vi "execute.vi"(10 "task token":refnum<class "null task token.lvclass">, 11 "noncancellable wait in":refnum<class "noncancellable wait.lvclass">) -> (3 "result":refnum<class "result.lvclass">)   [LabVIEW 2013, in "noncancellable wait.lvclass"]
uses:
  noncancellable wait.lvclass
  result/result.lvclass
  task token/null task token.lvclass
  action/action.lvclass/action.ctl
  action/action.lvclass
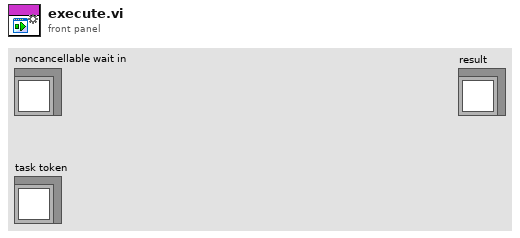
[diagram p1: front panel]
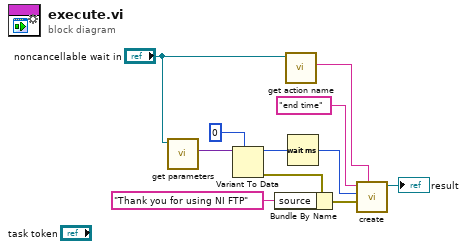
[diagram p0: block diagram]
diagram:
  n1 = call "get parameters.vi"("action in"="noncancellable wait in") -> ("parameters"=w11:variant)  [unwired: 9 in, 1 out]
  n2 = Variant To Data(type=u32 0 ("milliseconds to wait"), Variant=w11) -> (data=w2:u32, error out=w9:errorcluster)  [unwired: 1 in]
  n3 = Bundle By Name(cluster=w9, "source"="Thank you for using NI FTP") -> (w6:errorcluster)
  n4 = call "get action name.vi"("action in"="noncancellable wait in") -> ("action name"=w7:string)  [unwired: 9 in, 1 out]
  n5 = Wait (ms)(milliseconds to wait=w2) -> (millisecond timer value=w1:u32)
  n6 = call "create.vi"("generating action"=w7, "error"=w6, "data"=w1, "data ID"="end time") -> ("result out"=→"result":refnum<class "result.lvclass">)  [unwired: 7 in]
